vi "_100.vi"() -> ()   [LabVIEW 2020]
panel:
  out "o/p 3":i32[](array[numeric])
  out "o/p 4":i32[][](array[numeric])
  out "o/p 1":i32
  out "o/p 2":i32[](array[numeric])
  out "o/p 6":i32[](array[numeric])
  out "o/p 5":i32
  # "100th Day of My LabVIEW Journey"
  # "There are 3 rows with 4 colums in 2d array so the 3rd row will print in 2d array o/p . So the 1d array output was 3rd val will print"
  # "There are 3 rows in 2d array constant so the 2D array o/p was 3rd row will print."
  # "There are 3 rows with 4 colums in 2d array constant so the 3rd row will print. but in this new loop having only1 1d array so the o/p of Auto index o/p is 4\nSuppose if i connected 2D array with 3rows & 4columns connected to an array the o/p of Auto index is 3 why because the priority is rows"
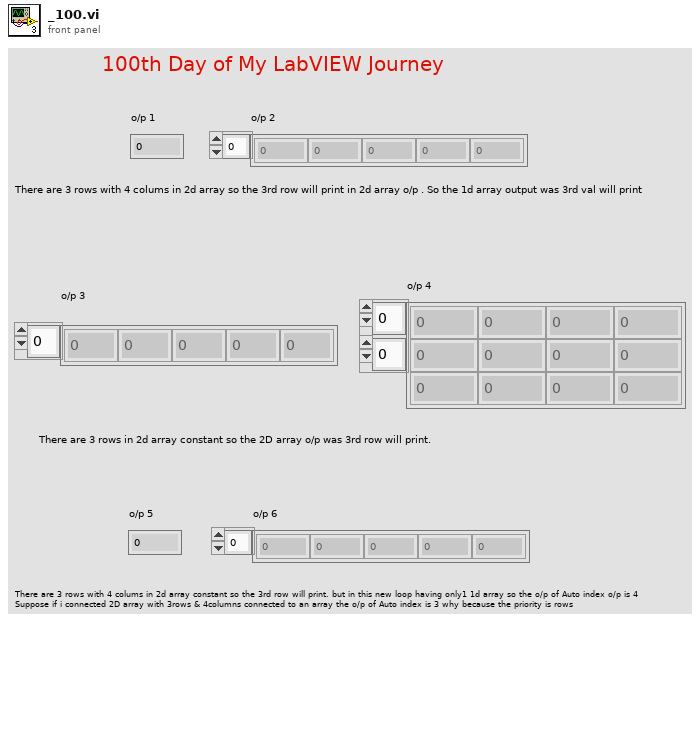
[diagram p1: front panel]
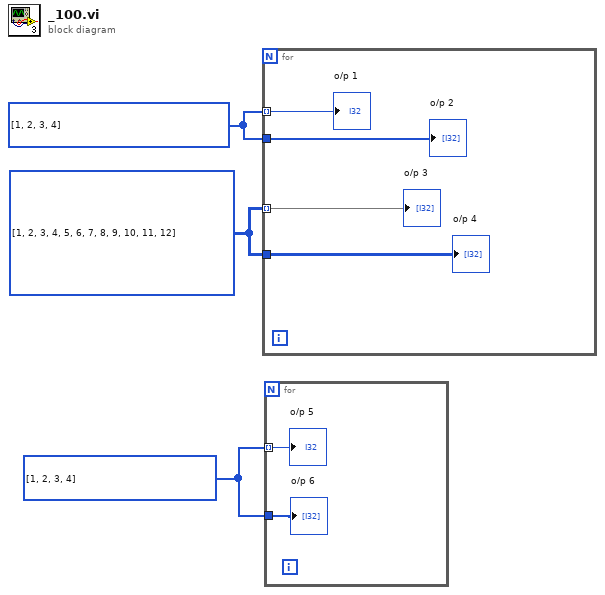
[diagram p0: block diagram]
diagram:
  w1 = i32[] [1, 2, 3, 4]
  w2 = i32[][] [[1, 2, 3, 4], [5, 6, 7, 8], [9, 10, 11, 12]]
  w3 = i32[] [1, 2, 3, 4]
  n1 = for {
    tunnel: w2 -> [w7] mode=indexing
    tunnel: w2 -> [w6]
    tunnel: w1 -> [w5] mode=indexing
    tunnel: w1 -> [w4]
    "o/p 3" <- w7
    "o/p 4" <- w6
    "o/p 1" <- w5
    "o/p 2" <- w4
  }
  n2 = for {
    tunnel: w3 -> [w9]
    tunnel: w3 -> [w8] mode=indexing
    "o/p 6" <- w9
    "o/p 5" <- w8
  }
